vi "Acquisition Message Loop.vi"(8 "error in (no error)":errorcluster, 9 "queue out":refnum<queue>, 10 "Data Notifier":refnum<notifier>, 11 "Message Queues":T1) -> (0 "error out":errorcluster)   [LabVIEW 2018, in "Acquisition.lvlib"]
doc: "Message loop for handling messages pertaining to the acquisition of data from the hardware."
uses:
  Acquisition.lvlib
  <vilib>/Utility/error.llb/Error Cluster From Error Code.vi
  support/Message Queue/Message Queue.lvlib
  Acquisition State.ctl
  support/Message Queue/Enqueue Message (Single).vi
  <vilib>/ErrorRing/Error Ring.xnode
  GlobalVariable/GlobalPowerByTime.vi
  GlobalVariable/Globalt0.vi
  GlobalVariable/GlobalLongueurOnde.vi
  GlobalVariable/GlobalDisconnected.vi
  GlobalVariable/GlobalPosXbyTime.vi
  GlobalVariable/GlobalPosYbyTime.vi
  GlobalVariable/GlobalProfileByTime.vi
  GlobalVariable/GlobalTimeStep.vi
  GlobalVariable/GlobalFirstRep.vi
  GlobalVariable/GlobalTensionByTime.vi
  GlobalVariable/GlobalTemperatureByTime.vi
  support/Message Queue/Message Cluster.ctl
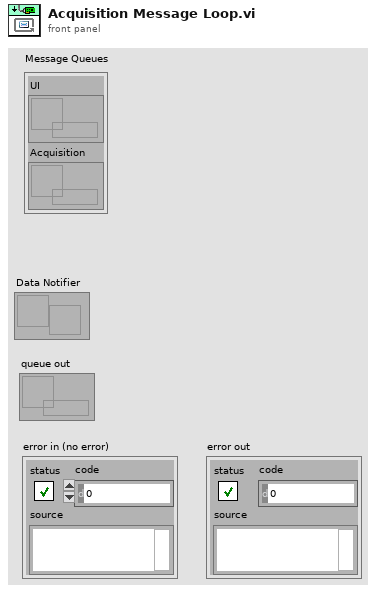
[diagram p1: front panel]
types:
  T1 = cluster{"UI":refnum<queue>, "Acquisition":refnum<queue>}
  T2 = typedef "Acquisition.lvlib/Acquisition State.ctl" = enum16{"Idle", "Acquiring"}
  T3 = enum16{"open", "replace", "create", "open or create", "replace or create", "replace or create with confirmation"}
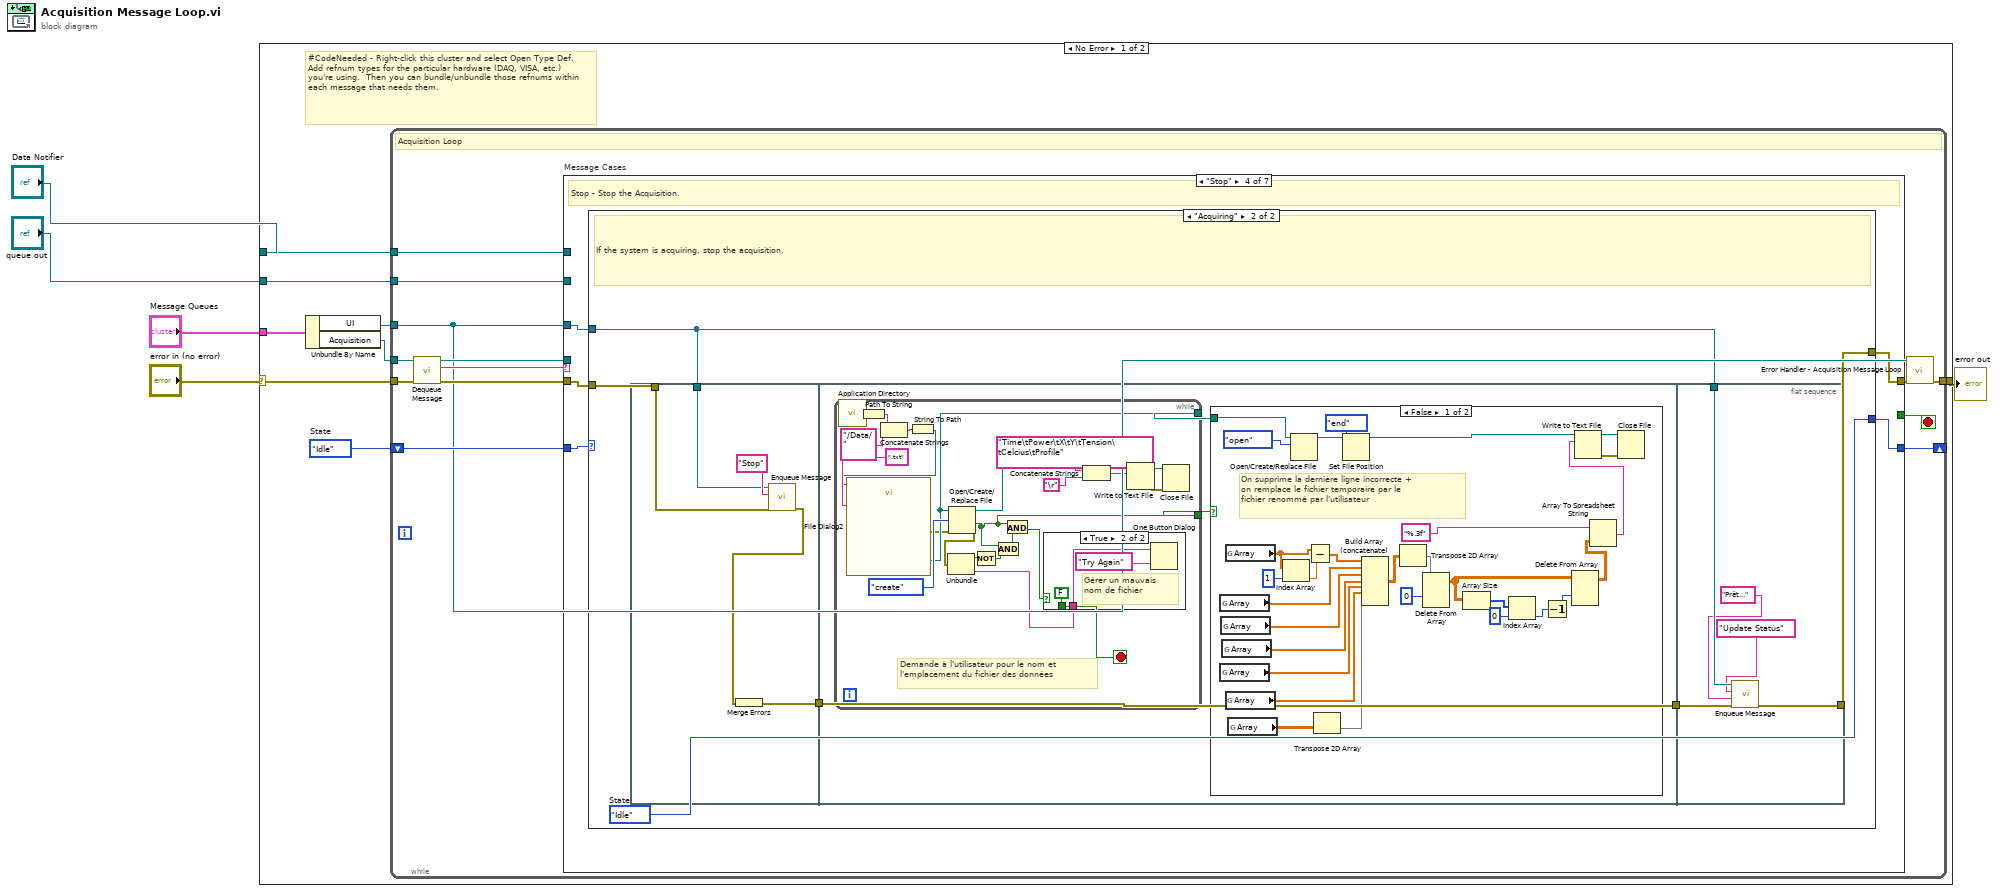
[diagram p0: block diagram]
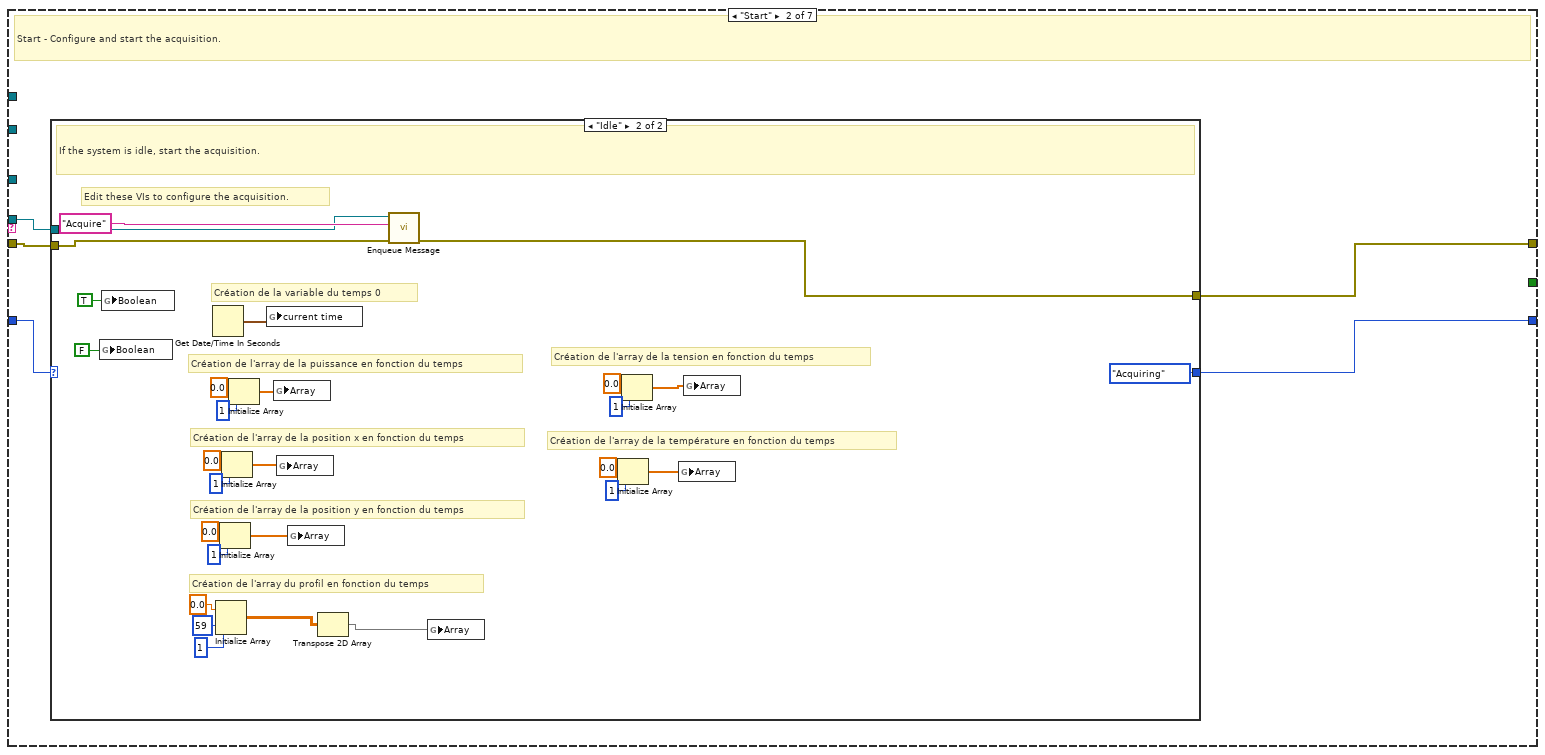
[diagram p3: hidden frame]
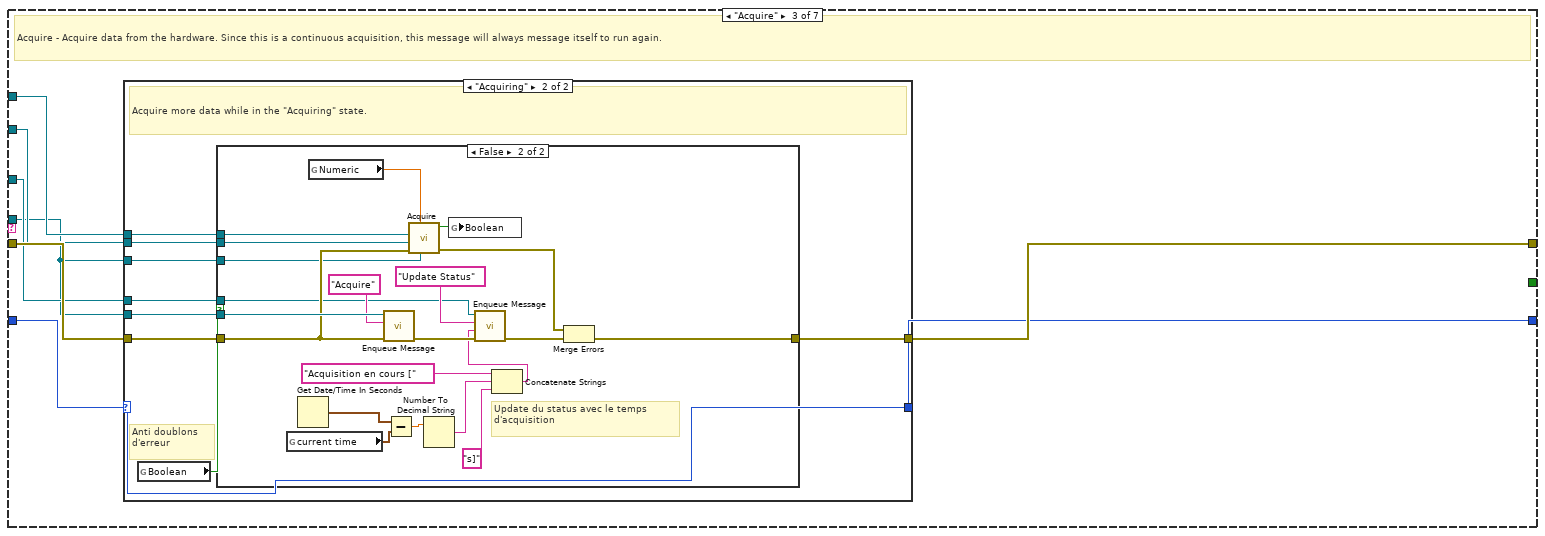
[diagram p5: hidden frame]
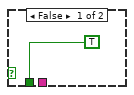
[diagram p10: hidden frame]
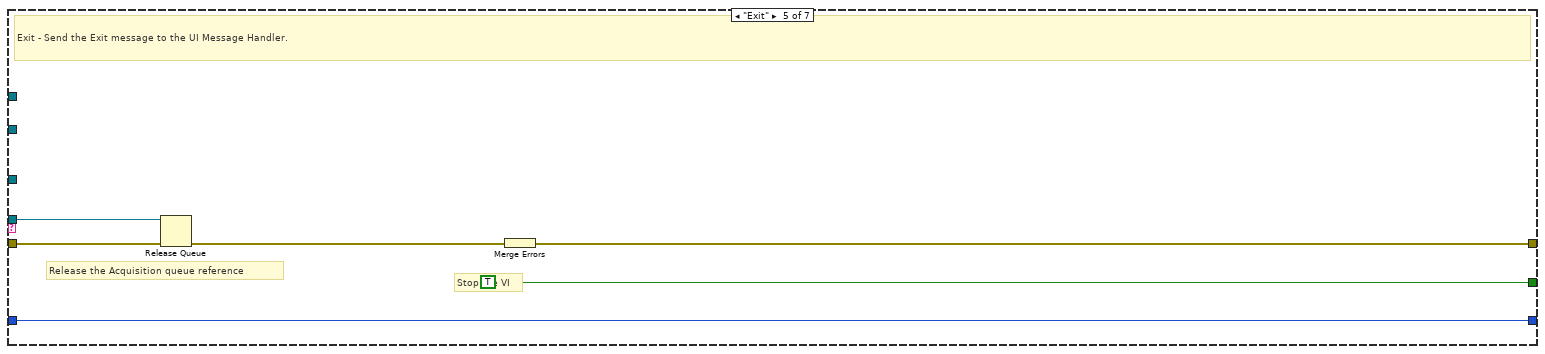
[diagram p11: hidden frame]
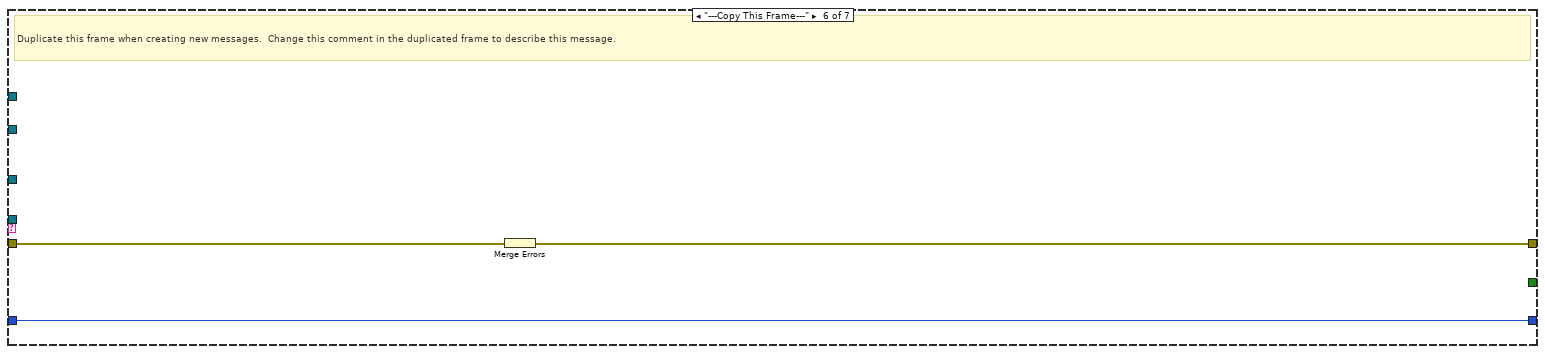
[diagram p12: hidden frame]
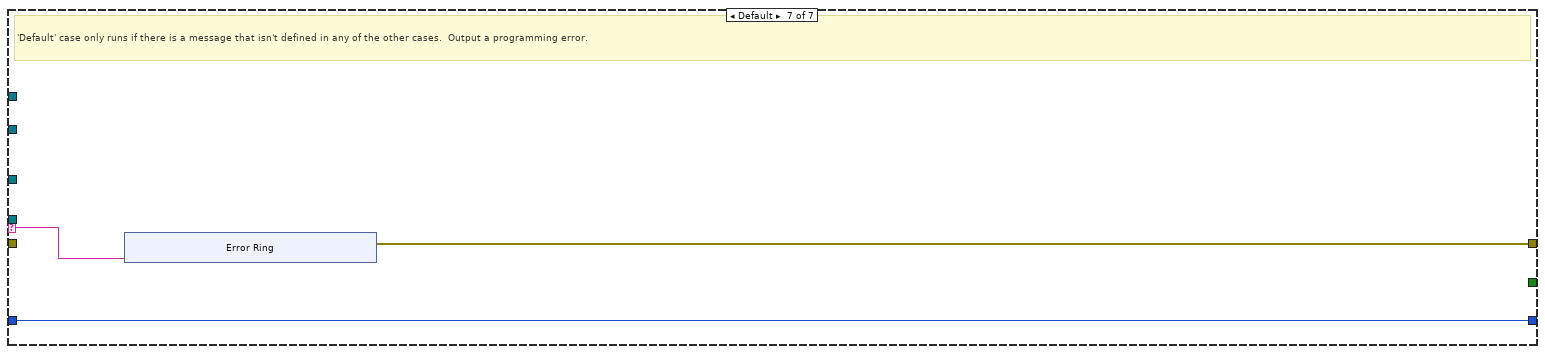
[diagram p13: hidden frame]
diagram:
  n1 = case shown="No Error" "error in (no error)" {
    selector: "error in (no error)" -> [w10 w206]
    tunnel: "Message Queues" -> [w13 _]
    tunnel: [w11 w206] -> w4
    tunnel: "Data Notifier" -> [w8 _]
    tunnel: "queue out" -> [w7 _]
    frame No Error {
      w6 = Acquisition_State."Idle"  # State
      # "#CodeNeeded - Right-click this cluster and select Open Type Def.  Add refnum types for the particular hardware (DAQ, VISA, etc.) you're using.  Then you can bundle/unbundle those refnums within each message that needs them."
      n2 = Unbundle By Name(w13) -> ("UI"=w9:refnum<queue>, "Acquisition"=w12:refnum<queue>)
      n3 = while {
        tunnel: w12 -> [w14]
        tunnel: w9 -> [w15]
        tunnel: w8 -> [w22]
        tunnel: w7 -> [w21]
        shift-right: [w19] -> _
        shift-left: w6 -> [w20]
        tunnel: w10 -> [w25]
        tunnel: [w18] -> w11
        stop <- w26 stop-if-true
        # "Acquisition Loop"
        n4 = call "Dequeue Message.vi"("error in (no error)"=w25, "Message Queue"=w14) -> ("error out"=w24:errorcluster, "Message"=w23:string, "dup Message Queue"=w16:refnum<queue>)  [unwired: 6 in, 1 out]
        n5 = case "Message Cases" shown="\"Stop\"" w23 {
          selector: w23 -> [_ _ _ _ _ _ w196]
          tunnel: w16 -> [_ w31 w64 _ w188 _ _]
          tunnel: w24 -> [w28 w32 w70 w108 w190 w195 _]
          tunnel: [w28 w33 w71 w106 w191 w194 w197] -> w17
          tunnel: [_ _ _ _ TRUE _ _] -> w26
          tunnel: w15 -> [_ _ w65 w107 _ _ _]
          tunnel: w22 -> [_ _ w69 _ _ _ _]
          tunnel: w21 -> [_ _ w68 _ _ _ _]
          tunnel: w20 -> [w27 w29 w66 w109 w187 w193 w198]
          tunnel: [w27 w30 w67 w105 w187 w193 w198] -> w19
          frame "Initialize" {
            # "Initialize  - Initialize is currently a no-op.  The hardware initialization takes place in the 'Start' message."
          }
          frame "Start" {
            # "Start - Configure and start the acquisition."
            n6 = case shown="\"Idle\"" w29 {
              selector: w29 -> [w34 _]
              tunnel: [w35 w59] -> w33
              tunnel: w32 -> [w35 w63]
              tunnel: w31 -> [_ w60]
              tunnel: [w34 Acquisition_State."Acquiring" ("Acquisition State")] -> w30
              frame "Acquiring" {
                # "The system is already acquiring. Ignore the \"Start\" message."
              }
              frame "Idle" {
                # "Création de l'array de la température en fonction du temps"
                # "Création de l'array de la tension en fonction du temps"
                # "Création de la variable du temps 0"
                # "Création de l'array du profil en fonction du temps"
                # "Création de l'array de la position y en fonction du temps"
                # "Création de l'array de la position x en fonction du temps"
                # "Création de l'array de la puissance en fonction du temps"
                # "Edit these VIs to configure the acquisition."
                # "If the system is idle, start the acquisition."
                n7 = global write "GlobalDisconnected.vi" "Boolean"(FALSE) -> ()
                n8 = global write "GlobalFirstRep.vi" "Boolean"(TRUE ("Boolean")) -> ()
                n9 = Get Date/Time In Seconds() -> (seconds since 1Jan1904=w42:timestamp)
                n10 = Initialize Array(0.0, 59 ("dimension size"), 1 ("dimension size")) -> (w55:dbl[][])
                n11 = Initialize Array(0.0, 1) -> (w56:dbl[])
                n12 = Initialize Array(0.0, 1) -> (w57:dbl[])
                n13 = Initialize Array(0.0, 1) -> (w58:dbl[])
                n14 = global write "Globalt0.vi" "current time"(w42) -> ()
                n15 = global write "GlobalPowerByTime.vi" "Array"(w58) -> ()
                n16 = global write "GlobalPosXbyTime.vi" "Array"(w57) -> ()
                n17 = global write "GlobalPosYbyTime.vi" "Array"(w56) -> ()
                n18 = Transpose 2D Array(2D array=w55) -> (transposed array=w54:dbl[][])
                n19 = call-poly "Enqueue Message.vi"("error in (no error)"=w63, "Message"="Acquire", "Message Queue"=w60) -> ("error out"=w59:errorcluster)  [unwired: 7 in, 1 out]
                n20 = global write "GlobalProfileByTime.vi" "Array"(w54) -> ()
                n21 = Initialize Array(0.0, 1) -> (w36:dbl[])
                n22 = Initialize Array(0.0, 1) -> (w37:dbl[])
                n23 = global write "GlobalTemperatureByTime.vi" "Array"(w36) -> ()
                n24 = global write "GlobalTensionByTime.vi" "Array"(w37) -> ()
              }
            }
          }
          frame "Acquire" {
            # "Acquire - Acquire data from the hardware. Since this is a continuous acquisition, this message will always message itself to run again."
            n25 = case shown="\"Acquiring\"" w66 {
              selector: w66 -> [w72 w78]
              tunnel: [w73 w82] -> w71
              tunnel: w64 -> [_ w81]
              tunnel: w70 -> [w73 w77]
              tunnel: w69 -> [_ w80]
              tunnel: w68 -> [_ w79]
              tunnel: [w72 w78] -> w67
              tunnel: w65 -> [_ w76]
              tunnel: w64 -> [_ w75]
              frame "Idle" {
                # "Ignore \"Acquire\" messages when the acquisition is idle."
              }
              frame "Acquiring" {
                # "Anti doublons\nd'erreur"
                # "Acquire more data while in the \"Acquiring\" state."
                n26 = global read "GlobalDisconnected.vi" "Boolean"() -> (w74:bool)
                n27 = case shown="False" w74 {
                  tunnel: [w83 w104] -> w82
                  tunnel: w81 -> [_ w103]
                  tunnel: w80 -> [_ w100]
                  tunnel: w79 -> [_ w99]
                  tunnel: w77 -> [w83 w98]
                  tunnel: w76 -> [_ w87]
                  tunnel: w75 -> [_ w86]
                  frame True {
                  }
                  frame False {
                    # "Update du status avec le temps\nd'acquisition"
                    n28 = global read "Globalt0.vi" "current time"() -> (w93:timestamp)
                    n29 = Get Date/Time In Seconds() -> (seconds since 1Jan1904=w92:timestamp)
                    n30 = global read "GlobalLongueurOnde.vi" "Numeric"() -> (w85:dbl)
                    n31 = call-poly "Enqueue Message.vi"("error in (no error)"=w98, "Message"="Acquire", "Message Queue"=w103) -> ("error out"=w96:errorcluster)  [unwired: 7 in, 1 out]
                    n32 = Subtract(x=w92, y=w93) -> (x-y=w94:dbl)
                    n33 = call "Acquire.vi"("Acquisition"=w86, "Longueur d'onde"=w85, "error in (no error)"=w98, "Data Queue"=w99, "Data Notifier"=w100) -> ("error out"=w102:errorcluster, "Disconnected"=w84:bool)  [unwired: 5 in]
                    n34 = Number To Decimal String(number=w94) -> (decimal integer string=w91:string)  [unwired: 1 in]
                    n35 = global write "GlobalDisconnected.vi" "Boolean"(w84) -> ()
                    n36 = Concatenate Strings("Acquisition en cours [", w91, "s]" ("string")) -> (w89:string)
                    n37 = call-poly "Enqueue Message.vi"("error in (no error)"=w96, "Message Data"=w89, "Message"="Update Status", "Message Queue"=w87) -> ("error out"=w97:errorcluster)  [unwired: 6 in, 1 out]
                    n38 = Merge Errors(w102, w97) -> (w104:errorcluster)
                  }
                }
              }
            }
          }
          frame "Stop" {
            # "Stop - Stop the Acquisition."
            n39 = case shown="\"Acquiring\"" w109 {
              selector: w109 -> [w111 _]
              tunnel: w108 -> [w110 w116]
              tunnel: w107 -> [_ w112]
              tunnel: [w110 w115] -> w106
              tunnel: [w111 w114] -> w105
              frame "Idle" {
                # "The system is already idle. Ignore the \"Stop\" message."
              }
              frame "Acquiring" {
                w114 = Acquisition_State."Idle"  # State
                # "If the system is acquiring, stop the acquisition."
                n40 = flat-sequence {
                  tunnel: [w122] -> w117
                  tunnel: w112 -> [w119]
                  tunnel: w116 -> [w118]
                  tunnel: w117 -> [w124]
                  tunnel: [w124] -> w113
                  tunnel: [w185] -> w115
                  tunnel: w113 -> [w186]
                  tunnel: w112 -> [w184]
                  frame #0 {
                    n41 = call-poly "Enqueue Message.vi"("error in (no error)"=w118, "Message"="Stop", "Message Queue"=w119) -> ("error out"=w121:errorcluster)  [unwired: 7 in, 1 out]
                    n42 = Merge Errors(w121) -> (w122:errorcluster)
                  }
                  frame #1 {
                    n43 = while {
                      tunnel: [w172] -> w125
                      tunnel: [w162] -> w123
                      stop <- w168 stop-if-true
                      # "Demande à l'utilisateur pour le nom et\nl'emplacement du fichier des données"
                      n44 = call <vilib>:"Application Directory.vi"() -> ("Application Directory"=w175:path)
                      n45 = Path To String(path=w175) -> (string=w176:string)
                      n46 = Concatenate Strings(w176, "/Data/") -> (w177:string)
                      n47 = String To Path(string=w177) -> (path=w161:path)
                      n48 = call "File Dialog2"("start path"=w161, "pattern (all files)"=".txt") -> ("selected path"=w172:path, "error out"=w170:errorcluster)  [unwired: 10 in, 2 out]
                      n49 = Open/Create/Replace File(file path (use dialog)=w172, error in=w170, operation (0:open)=T3."create") -> (refnum out=w157:refnum<file>, cancelled=w162:bool, error out=w167:errorcluster)  [unwired: 3 in]
                      n50 = Unbundle(w167) -> ("status"=w166:bool, "source"=w169:string)  [unwired: 1 out]
                      n51 = Not(x=w166) -> (.not. x?=w165:bool)
                      n52 = And(x=w162, y=w165) -> (x .and. y?=w164:bool)
                      n53 = And(x=w162, y=w164) -> (x .and. y?=w163:bool)
                      n54 = case shown="True" w163 {
                        tunnel: w169 -> [_ w181]
                        tunnel: [TRUE FALSE] -> w168
                        frame False {
                        }
                        frame True {
                          # "Gérer un mauvais \nnom de fichier"
                          n55 = One Button Dialog(message=w181, button name ("OK")="Try Again") -> ()  [unwired: 1 out]
                        }
                      }
                      n56 = Concatenate Strings("Time\tPower\tX\tY\tTension\tCelcius\tProfile", "\r") -> (w160:string)
                      n57 = Write to Text File(file (use dialog)=w157, text=w160) -> (refnum out=w156:refnum<file>, error out=w155:errorcluster)  [unwired: 2 in, 1 out]
                      n58 = Close File(refnum=w156, error in=w155) -> ()  [unwired: 2 out]
                    }
                    n59 = case shown="False" w123 {
                      tunnel: w125 -> [w148 _]
                      frame False {
                        # "On supprime la dernière ligne incorrecte + \non remplace le fichier temporaire par le \nfichier renommé par l'utilisateur"
                        n60 = global read "GlobalPowerByTime.vi" "Array"() -> (w147:dbl[])
                        n61 = global read "GlobalTensionByTime.vi" "Array"() -> (w127:dbl[])
                        n62 = global read "GlobalPosXbyTime.vi" "Array"() -> (w146:dbl[])
                        n63 = global read "GlobalPosYbyTime.vi" "Array"() -> (w145:dbl[])
                        n64 = global read "GlobalTimeStep.vi" "Array"() -> (w135:dbl[])
                        n65 = global read "GlobalTemperatureByTime.vi" "Array"() -> (w126:dbl[])
                        n66 = global read "GlobalProfileByTime.vi" "Array"() -> (w143:dbl[][])
                        n67 = Index Array(array=w135, index=1) -> (element=w136:dbl)
                        n68 = Open/Create/Replace File(file path (use dialog)=w148, operation (0:open)=T3."open") -> (refnum out=w152:refnum<file>)  [unwired: 4 in, 2 out]
                        n69 = Subtract(x=w135, y=w136) -> (x-y=w134:dbl[])
                        n70 = Transpose 2D Array(2D array=w143) -> (transposed array=w142:dbl[][])
                        n71 = Set File Position(refnum=w152, from (0:start)=enum16{"start", "end", "current"}."end") -> (refnum out=w154:refnum<file>)  [unwired: 2 in, 1 out]
                        n72 = Build Array (concatenate)(w134, w147, w146, w145, w127, w126, w142) -> (w144:dbl[][])
                        n73 = Transpose 2D Array(2D array=w144) -> (transposed array=w138:dbl[][])
                        n74 = Delete From Array(array=w138, index (row)=0) -> (array with subset deleted=w129:dbl[][])  [unwired: 2 in, 1 out]
                        n75 = Array Size(array=w129) -> (size(s)=w133:i32[])
                        n76 = Index Array(array=w133, index=0) -> (element=w131:i32)
                        n77 = Decrement(x=w131) -> (x-1=w130:i32)
                        n78 = Delete From Array(array=w129, index (row)=w130) -> (array with subset deleted=w128:dbl[][])  [unwired: 2 in, 1 out]
                        n79 = Array To Spreadsheet String(array=w128, 3:"%.3f" ("format string")) -> (spreadsheet string=w153:string)  [unwired: 1 in]
                        n80 = Write to Text File(file (use dialog)=w154, text=w153) -> (refnum out=w141:refnum<file>, error out=w140:errorcluster)  [unwired: 2 in, 1 out]
                        n81 = Close File(refnum=w141, error in=w140) -> ()  [unwired: 2 out]
                      }
                      frame True {
                      }
                    }
                  }
                  frame #2 {
                    n82 = call-poly "Enqueue Message.vi"("error in (no error)"=w186, "Message Data"="Prêt...", "Message"="Update Status", "Message Queue"=w184) -> ("error out"=w185:errorcluster)  [unwired: 6 in, 1 out]
                  }
                }
              }
            }
          }
          frame "Exit" {
            # "Release the Acquisition queue reference"
            # "Stop the VI"
            # "Exit - Send the Exit message to the UI Message Handler."
            n83 = Release Queue(queue=w188, error in (no error)=w190) -> (error out=w189:errorcluster)  [unwired: 1 in, 2 out]
            n84 = Merge Errors(w189) -> (w191:errorcluster)
          }
          frame "---Copy This Frame---" {
            # "Duplicate this frame when creating new messages.  Change this comment in the duplicated frame to describe this message."
            n85 = Merge Errors(w195) -> (w194:errorcluster)
          }
          frame Default {
            # "'Default' case only runs if there is a message that isn't defined in any of the other cases.  Output a programming error."
            n86 = xnode "Error Ring"("parameter 0"=w196) -> ("error out"=w197:errorcluster)
          }
        }
        n87 = call "Error Handler - Acquisition Message Loop.vi"("error in (no error)"=w17, "Message Queue"=w15) -> ("dup error in"=w18:errorcluster)  [unwired: 8 in, 1 out]
      }
    }
    frame Error {
    }
  }
  "error out" <- w4
